vi "Overlay Particle Analysis Results.vi"(6 "Color":u32(colorbox)=16711680, 7 "Group":string, 8 "error in":errorcluster, 9 "Overlay":T1(ring), 10 "Particle Reports (Pixels)":T3(array[cluster]), 11 "Image":T2) -> (0 "error out":errorcluster, 3 "Image Out":T2)   [LabVIEW 2016]
doc: "Overlay targets at the location of the feature points in the specified colors."
uses:
  <vilib>/vision/Image Controls.llb/IMAQ Image.ctl
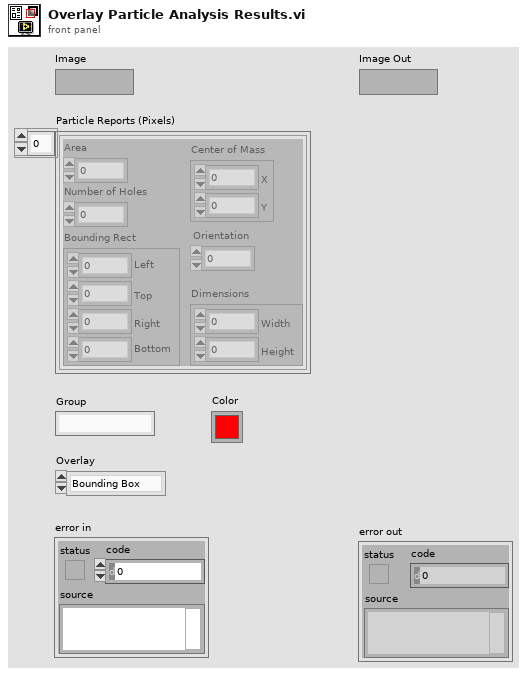
[diagram p1: front panel]
types:
  T1 = enum16{"Bounding Box", "ID Label", "Center of Mass"}
  T2 = typedef "IMAQ Image.ctl" = refnum<image>
  T3 = cluster{"Area":dbl, "Number of Holes":dbl, "Bounding Rect":cluster{"Left":dbl, "Top":dbl, "Right":dbl, "Bottom":dbl}, "Center of Mass":cluster{"X":dbl, "Y":dbl}, "Orientation":dbl, "Dimensions":cluster{"Width":dbl, "Height":dbl}}[]
  T4 = cluster{"Left":dbl, "Top":dbl, "Right":dbl, "Bottom":dbl}
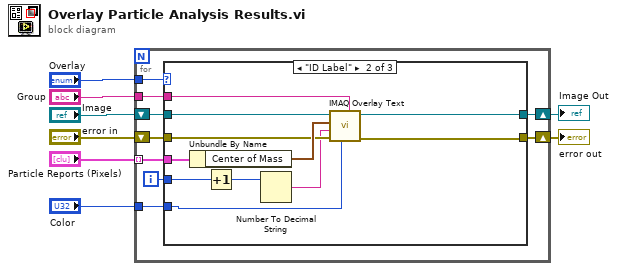
[diagram p0: block diagram]
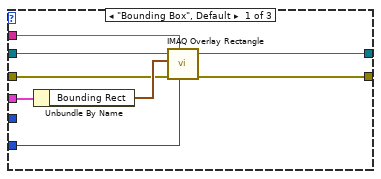
[diagram p2: hidden frame]
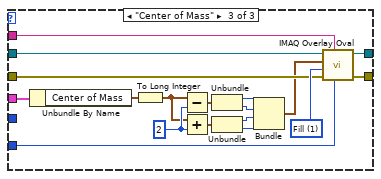
[diagram p3: hidden frame]
diagram:
  n1 = for {
    shift-right: [w10] -> w7
    shift-left: "Image" -> [w17]
    tunnel: "Particle Reports (Pixels)" -> [w15] mode=indexing
    tunnel: "Color" -> [w11]
    shift-right: [w12] -> w1
    shift-left: "error in" -> [w13]
    tunnel: "Overlay" -> [w16]
    tunnel: "Group" -> [w14]
    i -> [w9]
    n2 = case shown="\"ID Label\"" w16 {
      tunnel: w17 -> [w25 w32 w48]
      tunnel: w15 -> [w24 w36 w46]
      tunnel: w14 -> [w22 w35 w39]
      tunnel: w13 -> [w21 w33 w47]
      tunnel: [w20 w30 w41] -> w12
      tunnel: w11 -> [w19 w26 w38]
      tunnel: [w18 w29 w40] -> w10
      tunnel: w9 -> [_ w28 _]
      frame "Bounding Box", Default {
        n3 = Unbundle By Name(w24) -> ("Bounding Rect"=w23:T4)
        n4 = call "IMAQ Overlay Rectangle"("Color"=w19, "Group"=w22, "error in (no error)"=w21, "Rectangle"=w23, "Image"=w25) -> ("error out"=w20:errorcluster, "Image Out"=w18:T2)  [unwired: 5 in]
      }
      frame "ID Label" {
        n5 = Unbundle By Name(w36) -> ("Center of Mass"=w34:cluster{"X":dbl, "Y":dbl})
        n6 = Increment(x=w28) -> (x+1=w27:i32)
        n7 = Number To Decimal String(number=w27) -> (decimal integer string=w31:string)  [unwired: 1 in]
        n8 = call "IMAQ Overlay Text"("Group"=w35, "Text Color (black)"=w26, "error in (no error)"=w33, "String"=w31, "Origin"=w34, "Image"=w32) -> ("error out"=w30:errorcluster, "Image Out"=w29:T2)  [unwired: 4 in]
      }
      frame "Center of Mass" {
        w54 = u32 1 items=["Frame", "Fill"] ("Drawing Mode (Frame)")
        w49 = 2
        n9 = Unbundle By Name(w46) -> ("Center of Mass"=w43:cluster{"X":dbl, "Y":dbl})
        n10 = To Long Integer(number=w43) -> (32bit integer=w37:cluster{"X":i32, "Y":i32})
        n11 = Subtract(x=w37, y=w49) -> (x-y=w45:cluster{"X":i32, "Y":i32})
        n12 = Add(x=w37, y=w49) -> (x+y=w44:cluster{"X":i32, "Y":i32})
        n13 = Unbundle(w45) -> ("X"=w50:i32, "Y"=w51:i32)
        n14 = Unbundle(w44) -> ("X"=w52:i32, "Y"=w53:i32)
        n15 = Bundle("X"=w50, "Y"=w51, "X"=w52, "Y"=w53) -> (w42:cluster{"X":i32, "Y":i32, "X":i32, "Y":i32})  [unwired: 1 in]
        n16 = call "IMAQ Overlay Oval"("Color"=w38, "Group"=w39, "error in (no error)"=w47, "Drawing Mode (Frame)"=w54, "Bounding Rectangle"=w42, "Image"=w48) -> ("error out"=w41:errorcluster, "Image Out"=w40:T2)  [unwired: 4 in]
      }
    }
  }
  "Image Out" <- w7
  "error out" <- w1
